vi "Apply DSF Configuration.vi"(8 "error in (no error)":errorcluster, 10 "path":path, 11 "Item Ref in":T1 format="%.0x") -> (0 "error out":errorcluster)   [LabVIEW 2017, in "Data Sharing Framework System Explorer.lvlib"]
uses:
  Data Sharing Framework System Explorer.lvlib
  <vilib>/NI Veristand/Custom Device API/Custom Device Item Ref.ctl
  Engine/DSF Core.lvlibp/Classes/Configuration/Read All Plugin IDs.vi
  <vilib>/NI Veristand/Custom Device API/Custom Device API.lvlib
  Engine/DSF Core.lvlibp/Classes/Configuration/Configuration Session.lvclass
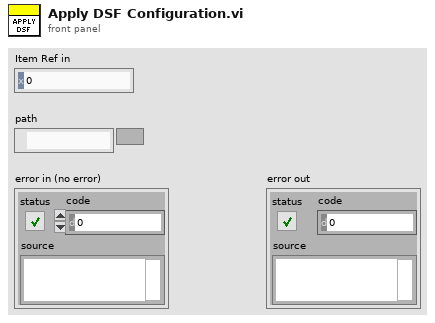
[diagram p1: front panel]
types:
  T1 = typedef "Custom Device API.lvlib/Custom Device Item Ref.ctl" = u64
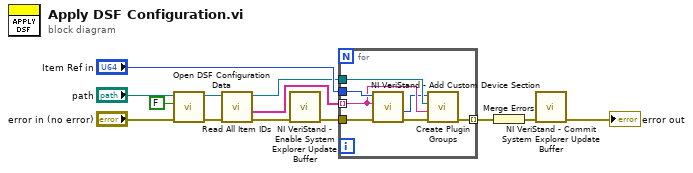
[diagram p0: block diagram]
diagram:
  n1 = call "Open DSF Configuration Data.vi"("error in (no error)"="error in (no error)", "create file if necessary (T)"=FALSE, "dsf configuration file path"="path") -> ("error out"=w5:errorcluster, "Configuration Session"=w6:refnum<class "Configuration Session.lvclass">)  [unwired: 4 in, 3 out]
  n2 = call-poly "Read All Item IDs.vi"("error in (no error)"=w5, "Configuration Session in"=w6) -> ("error out"=w2:errorcluster, "Plugin IDs"=w3:string[], "Configuration Session out"=w4:refnum<class "Configuration Session.lvclass">)  [unwired: 7 in]
  n3 = call <vilib>:"NI VeriStand - Enable System Explorer Update Buffer.vi"("error in (no error)"=w2) -> ("error out"=w7:errorcluster)  [unwired: 10 in]
  n4 = for {
    tunnel: w3 -> [w15] mode=indexing
    tunnel: "Item Ref in" -> [w20]
    tunnel: w7 -> [w19]
    tunnel: [w16] -> w9 mode=indexing
    tunnel: w4 -> [w18]
    n5 = call <vilib>:"NI VeriStand - Add Custom Device Section.vi"("error in (no error)"=w19, "Section Name"=w15, "Parent Ref in"=w20) -> ("error out"=w17:errorcluster, "Section Ptr"=w14:T1)  [unwired: 5 in, 2 out]
    n6 = call "Create Plugin Groups.vi"("error in (no error)"=w17, "String"=w15, "dsf refnum in"=w18, "Section Ptr"=w14) -> ("error out"=w16:errorcluster)  [unwired: 7 in]
  }
  n7 = Merge Errors(w9) -> (w8:errorcluster)
  n8 = call <vilib>:"NI VeriStand - Commit System Explorer Update Buffer.vi"("error in (no error)"=w8) -> ("error out"=→"error out":errorcluster)  [unwired: 10 in]
